vi "Write Ch 01.vi"(8 "error in":errorcluster, 10 "Producer Ch 01":T1, 11 "Chiller Cluster - 1 Channel.lvclass":refnum<class "Climate Chamber Cluster - 1 Channel.lvclass">) -> (0 "error out":errorcluster, 3 "output cluster":refnum<class "Climate Chamber Cluster - 1 Channel.lvclass">)   [LabVIEW 2023, in "Climate Chamber Cluster - 1 Channel.lvclass"]
uses:
  Climate Chamber Cluster - 1 Channel.lvclass
  Climate Chamber Cluster - 1 Channel.lvclass/Climate Chamber Cluster - 1 Channel.ctl
  d6de19df-c9e2-43fa-9ac5-572fde5e59f3.vi
  d6de19df-c9e2-43fa-9ac5-572fde5e59f3.vi/4bc1c15b-36ab-481f-b8dd-c64075ce723a.vi
  d6de19df-c9e2-43fa-9ac5-572fde5e59f3.vi/d83cb72b-7713-41fc-a3d1-682de79cf574.vi
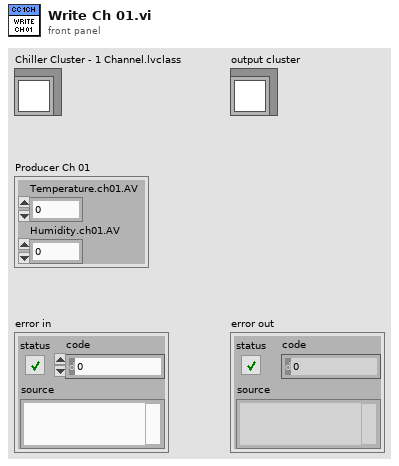
[diagram p1: front panel]
types:
  T1 = cluster{"Temperature.ch01.AV":dbl, "Humidity.ch01.AV":dbl}
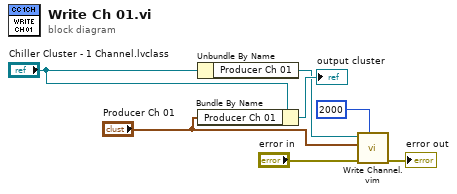
[diagram p0: block diagram]
diagram:
  n1 = Unbundle By Name("Chiller Cluster - 1 Channel.lvclass") -> ("Producer Ch 01"=w5:refnum<k21>)
  n2 = Bundle By Name(cluster="Chiller Cluster - 1 Channel.lvclass", "Producer Ch 01"="Producer Ch 01") -> (→"output cluster":refnum<class "Climate Chamber Cluster - 1 Channel.lvclass">)
  n3 = call "Write Channel.vim"("Timeout (ms)"=2000, "error in"="error in", "Data in"="Producer Ch 01", "ADAS HIL Channel in"=w5) -> ("error out"=→"error out":errorcluster)  [unwired: 5 in, 2 out]
